vi "CTRE_Phoenix_MotorController_Get_Enhanced.vi"   [LabVIEW 2019]
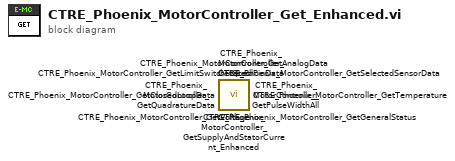
[diagram p0: block diagram]
diagram:
  n1 = call <vilib>:"CTRE_Phoenix_MotorController_GetSupplyAndStatorCurrent_Enhanced.vi"() -> ()  [unwired: 12 in, 4 out]
  n2 = call <vilib>:"CTRE_Phoenix_MotorController_GetQuadPinData.vi"() -> ()  [unwired: 11 in, 5 out]
  n3 = call <vilib>:"CTRE_Phoenix_MotorController_GetQuadratureData.vi"() -> ()  [unwired: 12 in, 4 out]
  n4 = call <vilib>:"CTRE_Phoenix_MotorController_GetPulseWidthAll.vi"() -> ()  [unwired: 10 in, 6 out]
  n5 = call <vilib>:"CTRE_Phoenix_MotorController_GetLimitSwitchStates.vi"() -> ()  [unwired: 12 in, 4 out]
  n6 = call <vilib>:"CTRE_Phoenix_MotorController_GetAnalogData.vi"() -> ()  [unwired: 11 in, 5 out]
  n7 = call <vilib>:"CTRE_Phoenix_MotorController_GetGeneralStatus.vi"() -> ()  [unwired: 10 in, 6 out]
  n8 = call <vilib>:"CTRE_Phoenix_MotorController_GetTemperature.vi"() -> ()  [unwired: 13 in, 3 out]
  n9 = call <vilib>:"CTRE_Phoenix_MotorController_GetClosedLoopData.vi"() -> ()  [unwired: 10 in, 6 out]
  n10 = call <vilib>:"CTRE_Phoenix_MotorController_GetSelectedSensorData.vi"() -> ()  [unwired: 12 in, 4 out]
  n11 = call <vilib>:"CTRE_Phoenix_MotorController_GetVoltage.vi"() -> ()  [unwired: 11 in, 5 out]
